vi "CDB to power dBm.vi"(11 "Y":cdb[](array[numeric])) -> (3 "Power dBm":dbl)   [LabVIEW 2020]
uses:
  <vilib>/Analysis/5stat.llb/RMS (CDB).vi
  <vilib>/Analysis/NI_AALPro.lvlib
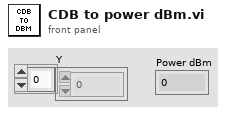
[diagram p1: front panel]
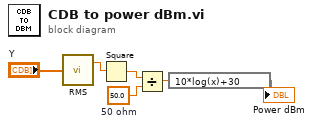
[diagram p0: block diagram]
diagram:
  w2 = 50.0  # 50 ohm
  n1 = call-poly <vilib>:"RMS.vi"("X"="Y") -> ("rms value"=w4:dbl)  [unwired: 1 out]
  n2 = Square(x=w4) -> (x^2=w3:dbl)
  n3 = Divide(x=w3, y=w2) -> (x/y=w5:dbl)
  n4 = expression code="10*log(x)+30"(w5) -> (→"Power dBm":dbl)
